vi "ConfigureSequence.vi"(0 "object in":refnum<class "Hamamatsu.lvclass">, 2 "Sequence Settings":T1={"Master Pulse Settings"={"Mode"=1, "Source"=1, "Interval"=1.0, "Burst"=0}, "Capture mode"=0, "Frames"=0, "Dcam Trigger Source"=1, "External Options"={"Polarity"=1, "Delay"=0.0}, "ExposureTime(ms)"=0.0} {"External Options"."Polarity" items=["Negative"=1, "Positive"=2]; "Dcam Trigger Source" items=["Internal"=1, "External"=2, "Software"=3, "Master Pulse"=4]; "Capture mode" items=["Snap", "Sequence"]; "Master Pulse Settings"."Source" items=["External"=1, "Software"=2]; "Master Pulse Settings"."Mode" items=["Continuous"=1, "Start"=2, "Burst"=3]}, 5 "error in (no error)":errorcluster) -> (14 "object out":refnum<class "Hamamatsu.lvclass">, 19 "error out":errorcluster)   [LabVIEW 2021, in "Hamamatsu.lvclass"]
uses:
  Hamamatsu.lvclass
  Hamamatsu.lvclass/Hamamatsu.ctl
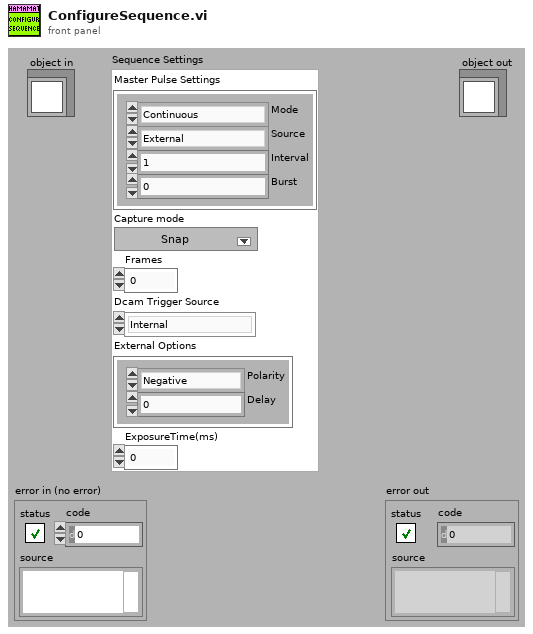
[diagram p1: front panel]
types:
  T1 = cluster{"Master Pulse Settings":cluster{"Mode":u32, "Source":u32, "Interval":dbl, "Burst":u32}, "Capture mode":i32, "Frames":i32, "Dcam Trigger Source":i32, "External Options":cluster{"Polarity":i32, "Delay":dbl}, "ExposureTime(ms)":dbl}
  T2 = cluster{"Mode":u32, "Source":u32, "Interval":dbl, "Burst":u32}
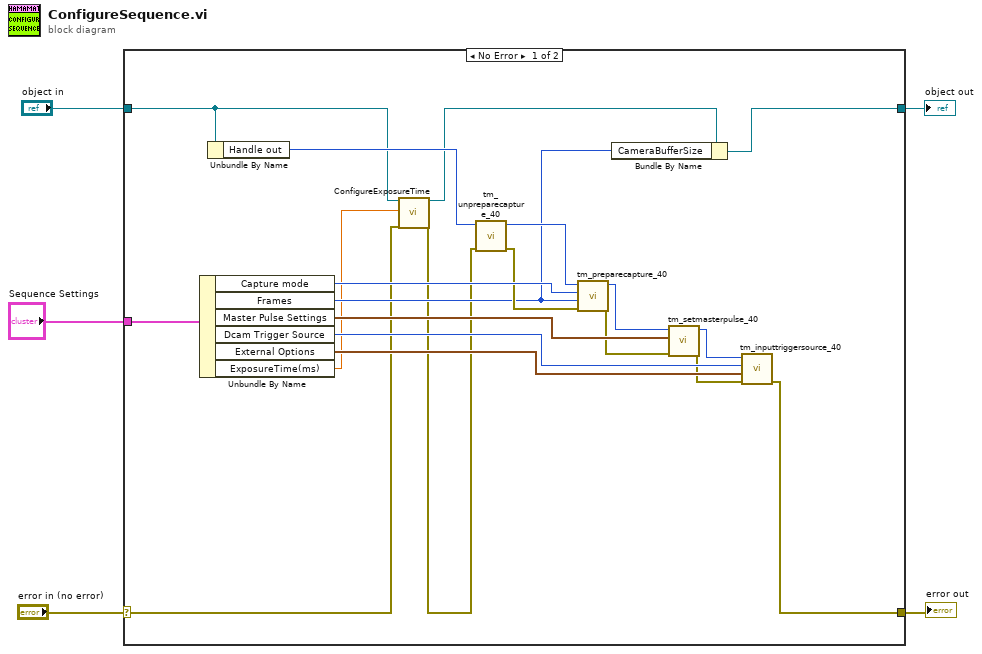
[diagram p0: block diagram]
diagram:
  n1 = case shown="No Error" "error in (no error)" {
    selector: "error in (no error)" -> [w8 w27]
    tunnel: [w16 w27] -> w4
    tunnel: [w12 w26] -> w2
    tunnel: "object in" -> [w9 w26]
    tunnel: "Sequence Settings" -> [w25 _]
    frame No Error {
      n2 = Unbundle By Name(w25) -> ("Capture mode"=w24:i32, "Frames"=w11:i32, "Master Pulse Settings"=w22:T2, "Dcam Trigger Source"=w19:i32, "External Options"=w18:cluster{"Polarity":i32, "Delay":dbl}, "ExposureTime(ms)"=w6:dbl)
      n3 = Unbundle By Name(w9) -> ("Handle out"=w15:u32)
      n4 = call-dynamic "ConfigureExposureTime.vi"("object in"=w9, "ExposureTime(ms)"=w6, "error in (no error)"=w8) -> ("object out"=w10:refnum<class "Hamamatsu.lvclass">, "error out"=w7:errorcluster)  [unwired: 15 in]
      n5 = call <userlib>:"tm_unpreparecapture_40.vi"("error in (no error)"=w7, "Handle in"=w15) -> ("error out"=w14:errorcluster, "Handle out"=w13:u32)  [unwired: 8 in]
      n6 = call <userlib>:"tm_preparecapture_40.vi"("error in (no error)"=w14, "Frames"=w11, "Capture mode"=w24, "Handle in"=w13) -> ("error out"=w21:errorcluster, "Handle out"=w23:u32)  [unwired: 4 in, 2 out]
      n7 = Bundle By Name(cluster=w10, "CameraBufferSize"=w11) -> (w12:refnum<class "Hamamatsu.lvclass">)
      n8 = call <userlib>:"tm_setmasterpulse_40.vi"("error in (no error)"=w21, "Parameters"=w22, "Handle in"=w23) -> ("error out"=w17:errorcluster, "Handle out"=w20:u32)  [unwired: 7 in]
      n9 = call <userlib>:"tm_inputtriggersource_40.vi"("error in (no error)"=w17, "External Options"=w18, "Source"=w19, "Handle in"=w20) -> ("error out"=w16:errorcluster)  [unwired: 6 in, 1 out]
    }
    frame Error {
    }
  }
  "error out" <- w4
  "object out" <- w2
